vi "Update.vi"(8 "error in (no error)":errorcluster, 10 "Message in":refnum<class "UpdateMessage.lvclass">, 11 "Cobolt in":refnum<class "Cobolt.lvclass">) -> (0 "error out":errorcluster, 3 "Cobolt out":refnum<class "Cobolt.lvclass">)   [LabVIEW 2012, in "Cobolt.lvclass"]
doc: "The update method processes the command 'update'. \n\nThe command 'update' is used for receiving new values to be set to the private data of the class. This could be seen as a public set method for setting new parameters to the private class data."
uses:
  Cobolt.lvclass
  <vilib>/Distrio/Murmex/UpdateMessage/UpdateMessage.lvclass
  Cobolt.lvclass/Cobolt.ctl
  <vilib>/Distrio/Murmex/Murmex/Murmex.lvclass
panel:
  # "This method is called when the UPDATE\ntrigger is sent. \n\nOverride this method when your component needs to\nrespond to this trigger. \n\nCall parent for proper implementation"
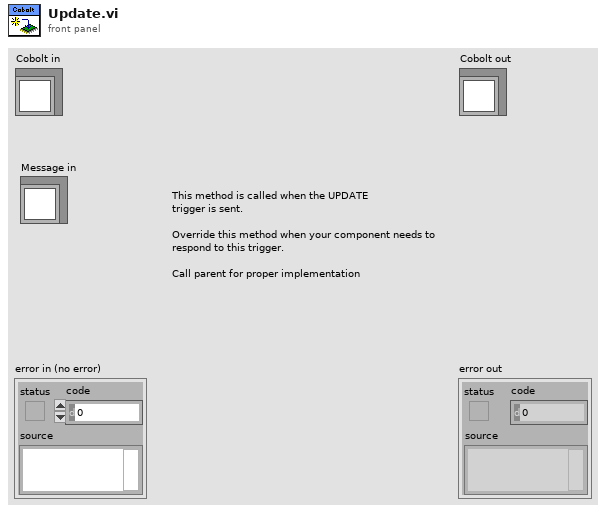
[diagram p1: front panel]
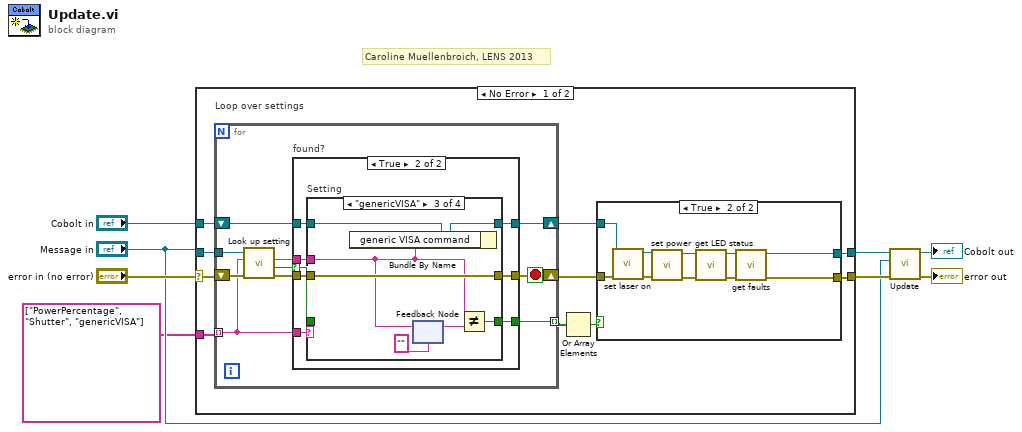
[diagram p0: block diagram]
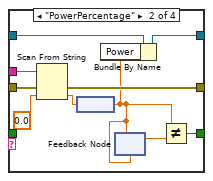
[diagram p5: hidden frame]
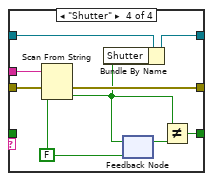
[diagram p6: hidden frame]
diagram:
  # "Caroline Muellenbroich, LENS 2013"
  n1 = case shown="No Error" "error in (no error)" {
    selector: "error in (no error)" -> [w18 w82]
    tunnel: "Message in" -> [w17 _]
    tunnel: "Cobolt in" -> [w16 w81]
    tunnel: [w11 w82] -> w6
    tunnel: [w9 w81] -> w2
    tunnel: string[] ["PowerPercentage", "Shutter", "genericVISA"] ("key chains") -> [w15 _]
    frame No Error {
      n2 = for "Loop over settings" {
        shift-right: [w33] -> w12
        shift-left: w18 -> [w40]
        tunnel: w17 -> [w39]
        shift-right: [w34] -> w10
        shift-left: w16 -> [w37]
        tunnel: w15 -> [w32] mode=indexing
        tunnel: [w31] -> w14 mode=indexing
        stop <- w33 stop-if-true
        n3 = call <vilib>:"Look up setting.vi"("error in (no error)"=w40, "tag name"=w32, "UpdateMessage in"=w39) -> ("error out"=w35:errorcluster, "found?"=w38:bool, "value"=w36:string)  [unwired: 5 in, 1 out]
        n4 = case "found?" shown="True" w38 {
          selector: w38 -> [w41 w45]
          tunnel: w37 -> [w43 w50]
          tunnel: w36 -> [_ w51]
          tunnel: w35 -> [w42 w49]
          tunnel: [w43 w48] -> w34
          tunnel: [w42 w47] -> w33
          tunnel: w32 -> [_ w46]
          tunnel: [w41 w44] -> w31
          frame False {
          }
          frame True {
            n5 = case "Setting" shown="\"genericVISA\"" w46 {
              tunnel: w51 -> [_ w60 w65 w78]
              tunnel: w50 -> [w54 w63 w71 w77]
              tunnel: w49 -> [w53 w64 w66 w80]
              tunnel: [w54 w62 w70 w76] -> w48
              tunnel: [w53 w61 w66 w79] -> w47
              tunnel: w45 -> [w52 _ _ _]
              tunnel: [w52 w58 w68 w74] -> w44
              frame Default {
              }
              frame "PowerPercentage" {
                n6 = Scan From String(input string=w60, error in=w64, default 1=0.0 ("Settings_cluster.Power")) -> (error out=w61:errorcluster, output 1=w57:dbl)  [unwired: 2 in, 2 out]
                n7 = node(w57) -> (w55:dbl[unit])
                n8 = Bundle By Name(cluster=w63, "Power"=w55) -> (w62:refnum<class "Cobolt.lvclass">)
                n9 = feedback-in #1(w55) -> ()
                n10 = feedback #1(w55) -> (w59:dbl[unit])
                n11 = Not Equal?(x=w55, y=w59) -> (x != y?=w58:bool)
              }
              frame "genericVISA" {
                n12 = Bundle By Name(cluster=w71, "generic VISA command"=w65) -> (w70:refnum<class "Cobolt.lvclass">)
                n13 = feedback-in #2(w65) -> ()
                n14 = feedback #2("" ("Run time cluster.generic VISA command")) -> (w69:string)
                n15 = Not Equal?(x=w65, y=w69) -> (x != y?=w68:bool)
              }
              frame "Shutter" {
                w75 = FALSE ("settings.Shutter")
                n16 = Scan From String(input string=w78, error in=w80, default 1=w75) -> (error out=w79:errorcluster, output 1=w72:bool)  [unwired: 2 in, 2 out]
                n17 = Bundle By Name(cluster=w77, "Shutter"=w72) -> (w76:refnum<class "Cobolt.lvclass">)
                n18 = feedback-in #3(w72) -> ()
                n19 = feedback #3(w75) -> (w73:bool)
                n20 = Not Equal?(x=w72, y=w73) -> (x != y?=w74:bool)
              }
            }
          }
        }
      }
      n21 = Or Array Elements(Boolean array=w14) -> (logical OR=w13:bool)
      n22 = case shown="True" w13 {
        tunnel: w12 -> [w20 w24]
        tunnel: [w20 w26] -> w11
        tunnel: w10 -> [w19 w22]
        tunnel: [w19 w25] -> w9
        frame False {
        }
        frame True {
          n23 = call-dynamic "set laser on.vi"("error in (no error)"=w24, "Cobolt in"=w22) -> ("error out"=w23:errorcluster, "Cobolt out"=w21:refnum<class "Cobolt.lvclass">)  [unwired: 8 in]
          n24 = call-dynamic "set power.vi"("error in (no error)"=w23, "Cobolt in"=w21) -> ("error out"=w29:errorcluster, "Cobolt out"=w30:refnum<class "Cobolt.lvclass">)  [unwired: 8 in]
          n25 = call-dynamic "get LED status.vi"("error in (no error)"=w29, "Cobolt in"=w30) -> ("error out"=w28:errorcluster, "Cobolt out"=w27:refnum<class "Cobolt.lvclass">)  [unwired: 4 in, 4 out]
          n26 = call-dynamic "get faults.vi"("error in (no error)"=w28, "Cobolt in"=w27) -> ("error out"=w26:errorcluster, "Cobolt out"=w25:refnum<class "Cobolt.lvclass">)  [unwired: 8 in]
        }
      }
    }
    frame Error {
    }
  }
  n27 = call-parent "Update.vi"("error in (no error)"=w6, "Message in"="Message in", "Murmex in"=w2) -> ("error out"=→"error out":errorcluster, "Murmex out"=→"Cobolt out":refnum<class "Cobolt.lvclass">)  [unwired: 7 in]
